vi "Set FPGA Reference.vi"(8 "Error In":errorcluster, 10 "FPGA VI Reference":T1, 11 "Display In":refnum<class "Neopixel - RT.lvclass">) -> (0 "Error Out":errorcluster, 3 "Display Out":refnum<class "Neopixel - RT.lvclass">)   [LabVIEW 2021, in "Neopixel - RT.lvclass"]
uses:
  Neopixel - RT.lvclass
  Public/Controls/FPGA Reference.ctl
  Neopixel - RT.lvclass/Neopixel - RT.ctl
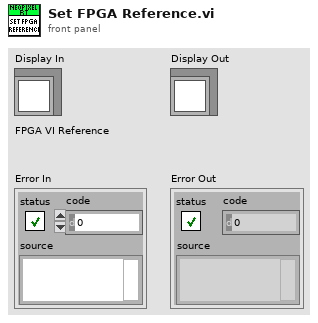
[diagram p1: front panel]
types:
  T1 = typedef "Neopixel - RT.lvclass/FPGA Reference.ctl" = refnum<k20>
  T2 = typedef "Neopixel - RT.lvclass/Data.ctl" = cluster{"FPGA VI Reference":T1, "RGB Gains":T3}
  T3 = typedef "Neopixel - RT.lvclass/RGB Gains.ctl" = cluster{"Red":sgl, "Green":sgl, "Blue":sgl}
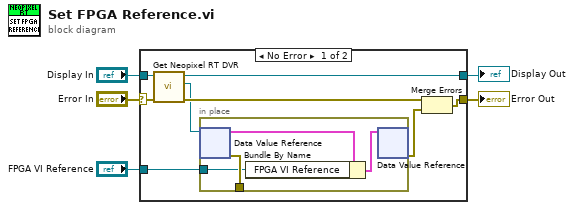
[diagram p0: block diagram]
diagram:
  n1 = case shown="No Error" "Error In" {
    selector: "Error In" -> [w10 w18]
    tunnel: [w12 w18] -> w1
    tunnel: [w7 w19] -> w2
    tunnel: "Display In" -> [w9 w19]
    tunnel: "FPGA VI Reference" -> [w11 _]
    frame No Error {
      n2 = call "Get Neopixel RT DVR.vi"("Error In"=w10, "Display In"=w9) -> ("Error Out"=w8:errorcluster, "DVR"=w6:refnum<data-value>, "Display Out"=w7:refnum<class "Neopixel - RT.lvclass">)  [unwired: 7 in]
      n3 = in-place {
        in-place-border: [w17] -> _
        in-place-border: w11 -> [w14]
        n4 = in-place-dvr #1(w6) -> (w16:T2, w17:errorcluster)
        n5 = Bundle By Name(cluster=w16, "FPGA VI Reference"=w14) -> (w15:T2)
        n6 = in-place-dvr #1(w15) -> (w13:errorcluster)  [unwired: 1 out]
      }
      n7 = Merge Errors(w8, w13) -> (w12:errorcluster)
    }
    frame Error {
    }
  }
  "Error Out" <- w1
  "Display Out" <- w2
